vi "LcWebView_PiePlot_Example.vi"() -> ()   [LabVIEW 2019, in "LcWebView.lvclass"]
doc: "Inject javascript arguments"
uses:
  LcWebView.lvclass
  ctrls/PlotType.ctl
  <vilib>/numeric/Random Number (Range) I64.vi
  ctrls/PiePlotOption.ctl
  Program Files/National Instruments/LabVIEW 2020/user.lib/_LabVIEWCommon/LcHTMLPlot/HTMLPlot_class/Controls/LegendPosition.ctl
  Program Files/National Instruments/LabVIEW 2020/user.lib/_LabVIEWCommon/LcHTMLPlot/HTMLPlot_class/HTMLPlot.lvclass
  ctrls/GenericPlotOption.ctl
  C:/Projects/WebView2/LcWebView/data/Microsoft.Web.WebView2.WinForms.dll
panel:
  out "BrowserProcessId":u32
  out "Source Change":string
  out "Status Message":string
  in  "stop":bool
  in  "Web":refnum<k24>(container)
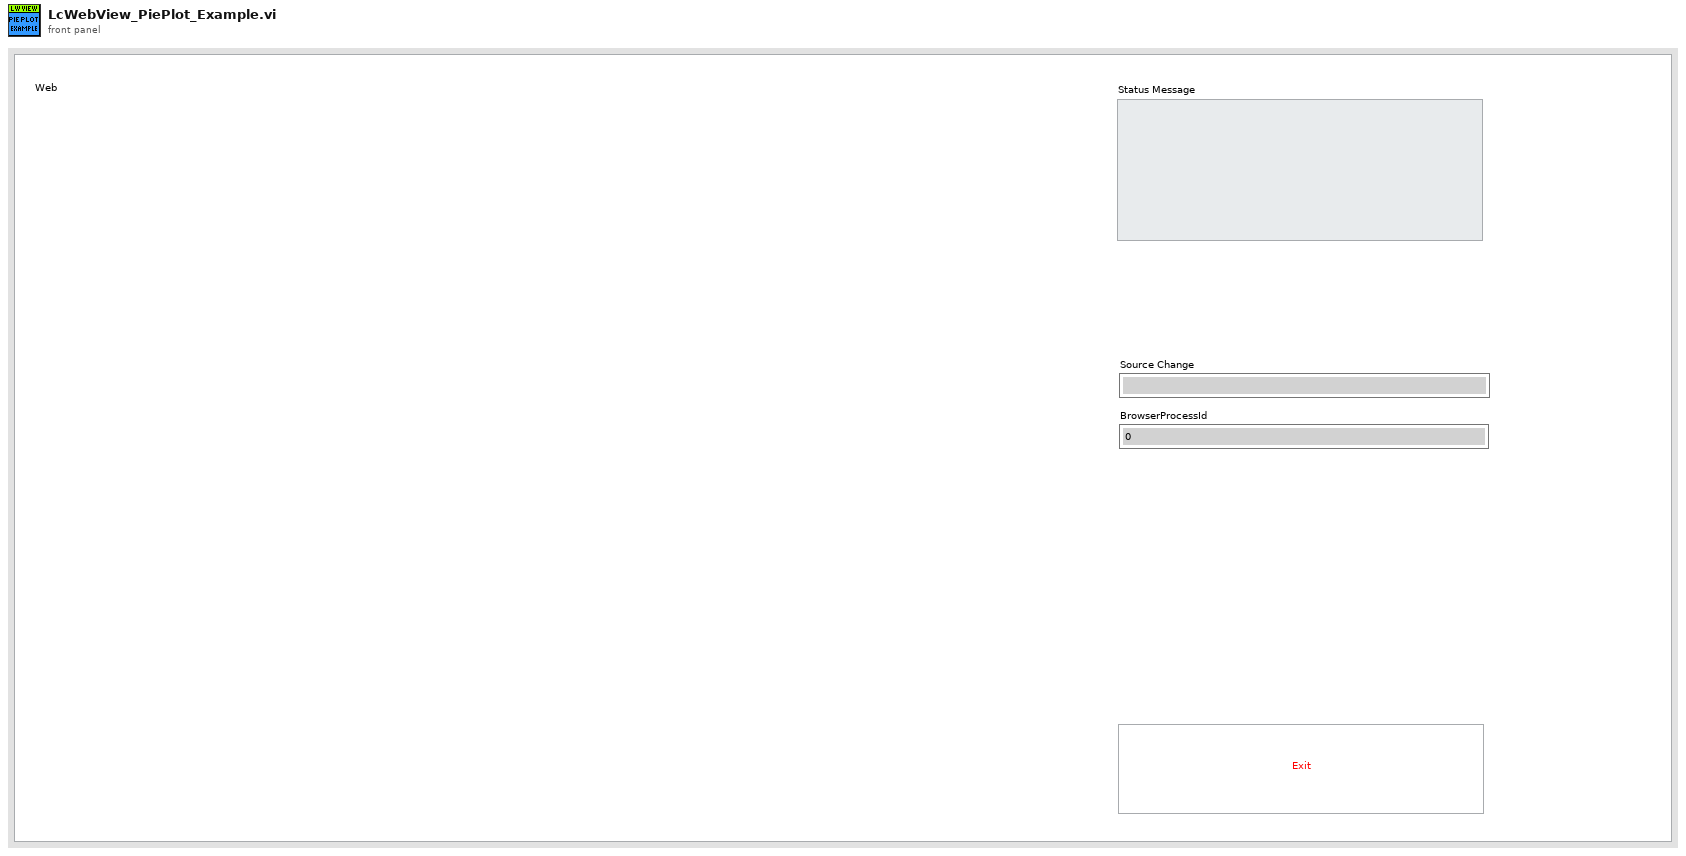
[diagram p1: front panel]
types:
  T1 = typedef "LcWebView.lvclass/GenericPlotOption.ctl" = cluster{"GraphTitle":string, "LegendDisplay":bool, "LegendPosition":T2}
  T2 = typedef "HTMLPlot.lvclass/LegendPosition.ctl" = enum16{"top", "right", "left", "bottom"}
  T3 = typedef "LcWebView.lvclass/PiePlotOption.ctl" = cluster{"cutoutPercentage":i32}
  T4 = typedef "LcWebView.lvclass/PlotType.ctl" = enum16{"bar", "line", "pie"}
  T5 = typedef "LcWebView.lvclass/WebViewDynamicEvents.ctl" = cluster{"Event Registration Ref":refnum<event-registration>, "Source event":refnum<user-event>}
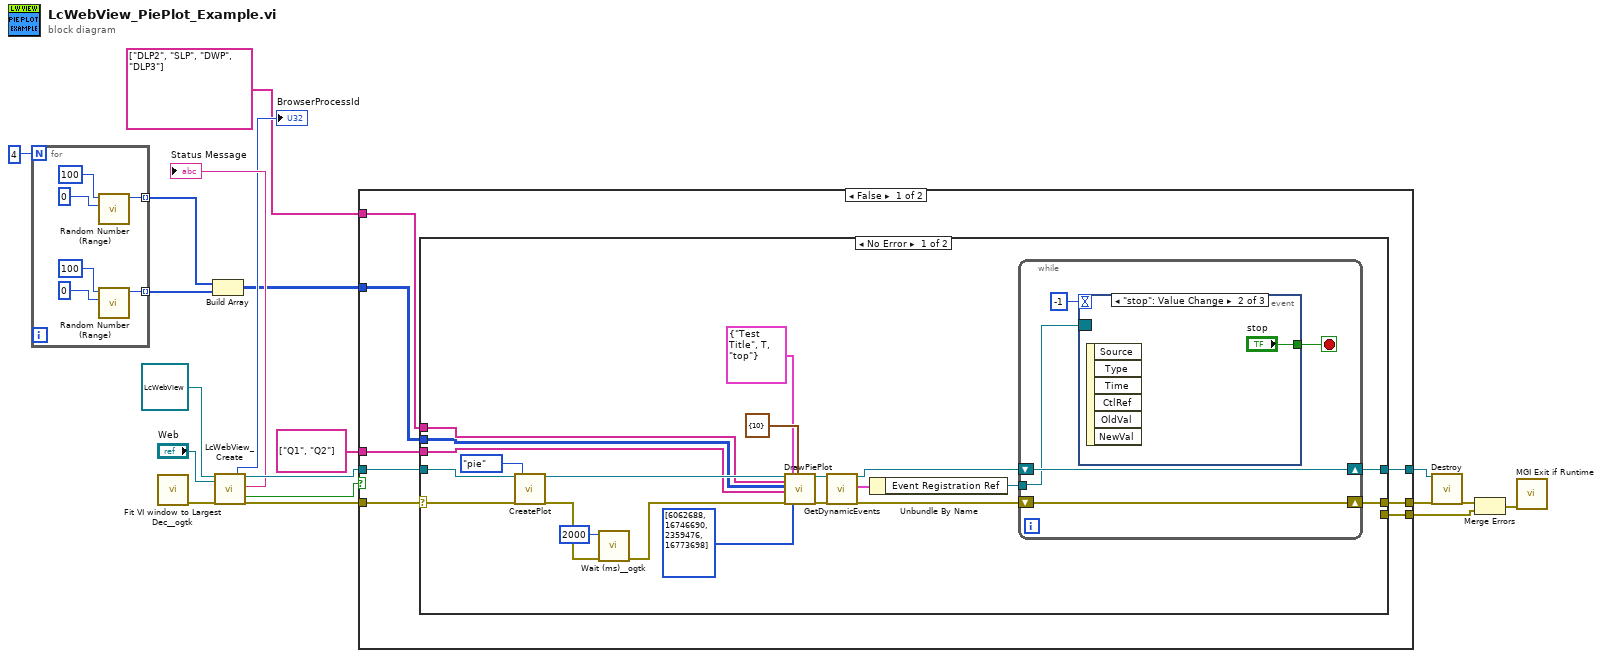
[diagram p0: block diagram]
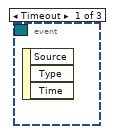
[diagram p2: hidden frame]
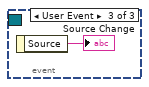
[diagram p3: hidden frame]
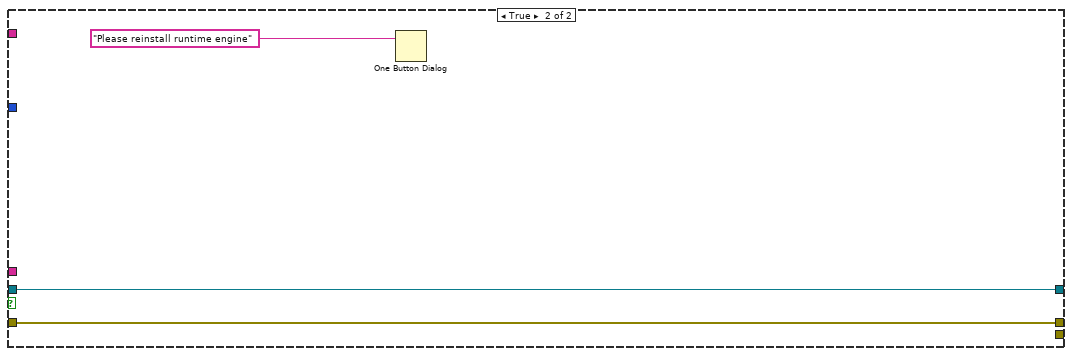
[diagram p5: hidden frame]
diagram:
  n1 = for {
    N: 4 -> [_]
    tunnel: [w21] -> w5 mode=indexing
    tunnel: [w20] -> w6 mode=indexing
    n2 = call-poly <vilib>:"Random Number (Range).vi"("lower bound (-100)"=i64 0, "upper bound (100)"=i64 100) -> ("number"=w21:i64)  [unwired: 9 in]
    n3 = call-poly <vilib>:"Random Number (Range).vi"("lower bound (-100)"=i64 0, "upper bound (100)"=i64 100) -> ("number"=w20:i64)  [unwired: 9 in]
  }
  n4 = call "Fit VI window to Largest Dec__ogtk.vi"() -> ("error out"=w9:errorcluster)  [unwired: 6 in, 1 out]
  n5 = Build Array(w5, w6) -> (w1:i64[][])
  n6 = call "LcWebView_Create.vi"("reference in"=refnum<class "LcWebView.lvclass"> refnum, "Webview container"="Web", "Error In"=w9) -> ("BrowserProcessId"=→"BrowserProcessId":u32, "reference out"=w17:refnum<class "LcWebView.lvclass">, "Status Message"=→"Status Message":string, "Reinstall Runtime"=w10:bool, "Error Out"=w16:errorcluster)  [unwired: 9 in, 3 out]
  n7 = case shown="False" w10 {
    tunnel: w17 -> [w33 w66]
    tunnel: w16 -> [w32 w65]
    tunnel: [w31 w66] -> w15
    tunnel: [w29 w65] -> w14
    tunnel: [w30 _] -> w11
    tunnel: string[] ["DLP2", "SLP", "DWP", "DLP3"] ("DatasetLabels") -> [w28 _]
    tunnel: string[] ["Q1", "Q2"] ("PiePlot.PlotLabels") -> [w27 _]
    tunnel: w1 -> [w26 _]
    frame False {
      n8 = case shown="No Error" w32 {
        selector: w32 -> [w51 w62]
        tunnel: w33 -> [w52 w63]
        tunnel: [w44 w63] -> w31
        tunnel: [w54 _] -> w29
        tunnel: [_ w62] -> w30
        tunnel: w28 -> [w41 _]
        tunnel: w27 -> [w40 _]
        tunnel: w26 -> [w39 _]
        frame No Error {
          n9 = call-dynamic "CreatePlot.vi"("reference in"=w52, "Error In"=w51, "PlotType"=PlotType."pie") -> ("reference out"=w49:refnum<class "LcWebView.lvclass">, "Error Out"=w50:errorcluster)  [unwired: 15 in]
          n10 = call "Wait (ms)__ogtk.vi"("error in (no error)"=w50, "milliseconds to wait"=u32 2000) -> ("error out"=w35:errorcluster)  [unwired: 8 in, 1 out]
          n11 = call-dynamic "DrawPiePlot.vi"("reference in"=w49, "PiePlot.PlotLabels"=w41, "PiePlot.Dataset"=w39, "PiePlot.DatasetLabels"=w40, "Error In"=w35, "GenericPlotOptions"=T1 {"GraphTitle"="Test Title", "LegendDisplay"=TRUE, "LegendPosition"=enum."top"}, "PiePlot.PlotColours"=u32[] [6062688, 16746690, 2359476, 16773698] ("PlotColours"), "PiePlotOptions"=T3 {"cutoutPercentage"=10}) -> ("reference out"=w48:refnum<class "LcWebView.lvclass">, "Error Out"=w47:errorcluster)  [unwired: 10 in]
          n12 = call-dynamic "GetDynamicEvents.vi"("reference in"=w48, "Error In"=w47) -> ("reference out"=w45:refnum<class "LcWebView.lvclass">, "DynamicEvents"=w43:T5, "Error Out"=w46:errorcluster)  [unwired: 15 in]
          n13 = Unbundle By Name(w43) -> ("Event Registration Ref"=w53:refnum<event-registration>)
          n14 = while {
            shift-right: [w59] -> w44
            shift-left: w45 -> [w59]
            shift-right: [w58] -> w54
            shift-left: w46 -> [w58]
            tunnel: w53 -> [w55]
            stop <- w56 stop-if-true
            n15 = event shown="[1] \"stop\": Value Change" {
              selector: w55 -> [_ _ _]
              dyn-events: _ -> [_ _ _]
              timeout: -1 -> [_ _ _]
              tunnel: [_ "stop" _] -> w56
              event Timeout {
                n16 = event-data() -> ()  [unwired: 1 in, 3 out]
              }
              event "stop": Value Change {
                n17 = event-data() -> ()  [unwired: 1 in, 6 out]
              }
              event User Event {
                n18 = event-data() -> ("Source"=→"Source Change":string)  [unwired: 1 in]
              }
            }
          }
        }
        frame Error {
        }
      }
    }
    frame True {
      n19 = One Button Dialog(message="Please reinstall runtime engine") -> ()  [unwired: 1 in, 1 out]
    }
  }
  n20 = call-dynamic "Destroy.vi"("reference in"=w15, "Error In"=w14) -> ("Error Out"=w13:errorcluster)  [unwired: 16 in, 1 out]
  n21 = Merge Errors(w13, w11) -> (w8:errorcluster)
  n22 = call "MGI Exit if Runtime.vi"("Error In (Dependency Only)"=w8) -> ()  [unwired: 11 in]
